vi "Generate BER Curve.vi"(4 "M-PSK":i32=4, 6 "Sample Step":dbl=0.3, 7 "Samples":i32=16, 9 "Message Bits":i32=2000, 10 "Synchronization Sequence":i32=20, 11 "Zero Pad":i32=16) -> (0 "error out":errorcluster, 3 "BER Curve":dbl[](array[numeric]))   [LabVIEW 2013]
uses:
  <vilib>/addons/Modulation/Digital/General/MT Generate Bits (Galois, PN Order).vi
  <vilib>/addons/Modulation/Digital/General/MT Generate PSK System Parameters(M).vi
  <vilib>/addons/Modulation/Digital/General/MT Generate PSK Synchronization Parameters (bit array).vi
  <vilib>/addons/Modulation/niDMT.lvlib
panel:
  out "O":bool[](array[boolean])
  out "I":bool[](array[boolean])
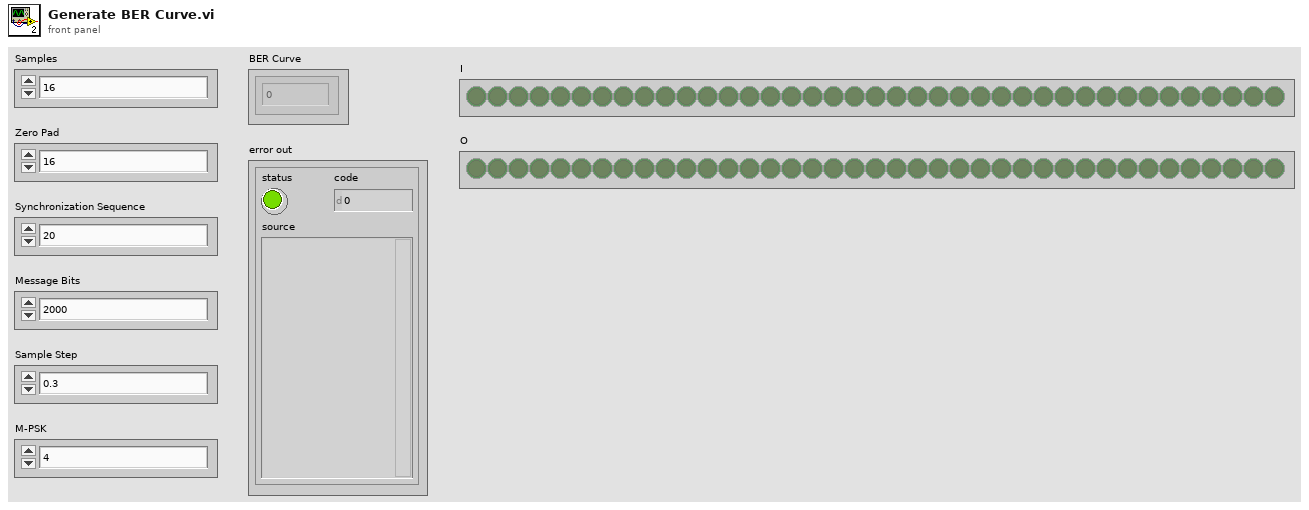
[diagram p1: front panel]
types:
  T1 = enum16{"FSK", "PSK", "QAM", "MSK", "PAM", "ASK", "CPM"}
  T2 = enum16{"none", "Raised Cosine", "Root Raised Cos", "Gaussian"}
  T3 = cluster{"samples per symbol (16)":i32, "symbol map":cdb[], "differential PSK":enum16{"disable", "enable"}, "PSK type":u16}
  T4 = typedef "niAMT.lvlib/Complex Data Waveform.ctl" = cluster{"t0":dbl, "dt":dbl, "Y":cdb[]}
  T5 = cluster{"expected sync location (symbols)":i32, "sync sequence":cdb[], "sync location uncertainty (symbols)":i32, "sync indent (symbols)":i32}
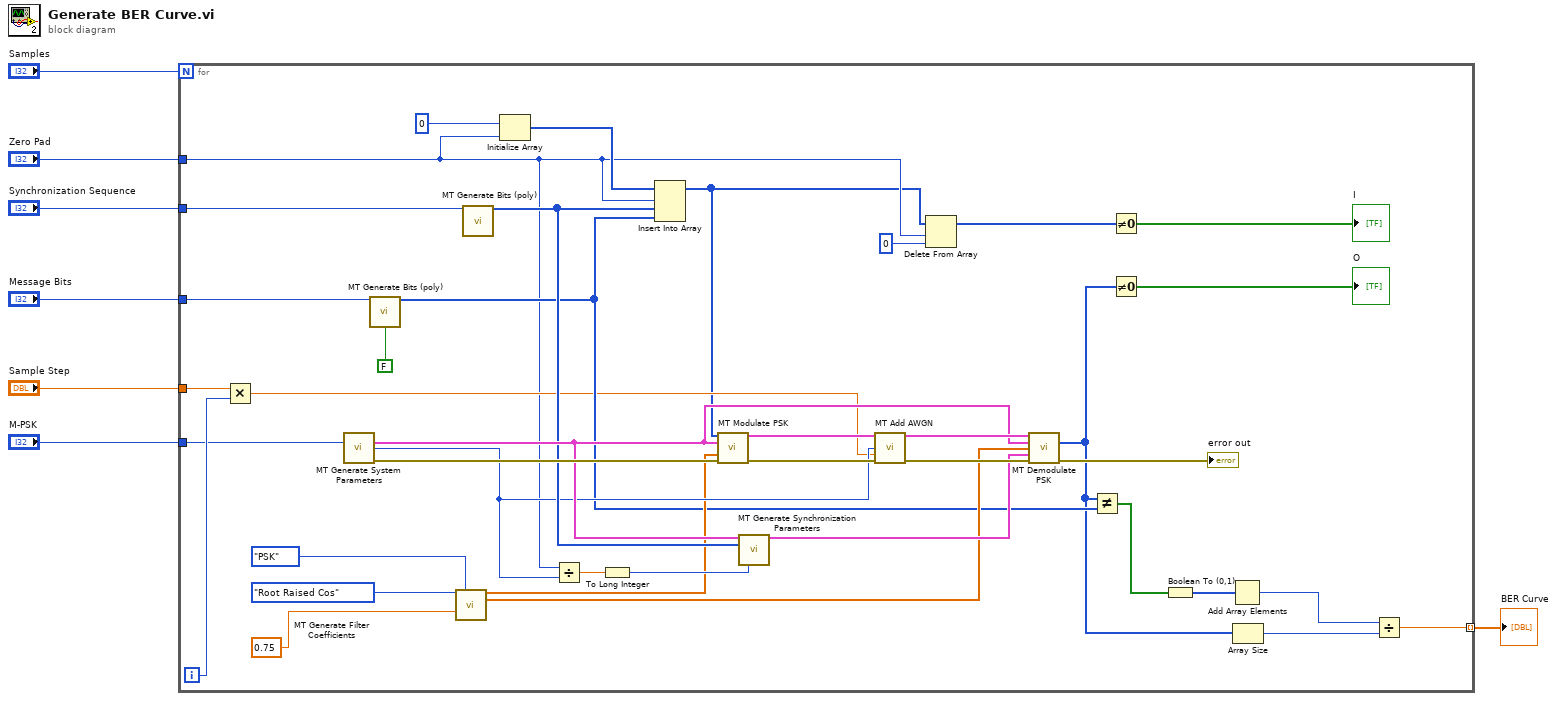
[diagram p0: block diagram]
diagram:
  n1 = for {
    N: "Samples" -> [_]
    tunnel: "Sample Step" -> [w20]
    tunnel: "Synchronization Sequence" -> [w19]
    tunnel: "Zero Pad" -> [w11]
    tunnel: "M-PSK" -> [w18]
    tunnel: [w17] -> w7 mode=indexing
    tunnel: "Message Bits" -> [w15]
    i -> [w21]
    n2 = Multiply(x=w20, y=w21) -> (x*y=w22:dbl)
    n3 = call-poly <vilib>:"MT Generate System Parameters.vi"("M-PSK (4)"=w18) -> ("PSK system parameters"=w38:T3, "bits per symbol"=w33:i32, "error out"=w43:errorcluster)  [unwired: 12 in]
    n4 = call-poly <vilib>:"MT Generate Bits (poly).vi"("total bits (128)"=w15, "reset? (T)"=FALSE) -> ("output bit stream"=w23:i8[])  [unwired: 11 in, 2 out]
    n5 = call <vilib>:"MT Generate Filter Coefficients.vi"("pulse shaping filter (none)"=T2."Root Raised Cos", "modulation type"=T1."PSK", "filter parameter"=0.75) -> ("pulse shaping filter coefficients"=w32:dbl[], "matched filter coefficients"=w31:dbl[])  [unwired: 10 in, 1 out]
    n6 = call-poly <vilib>:"MT Generate Bits (poly).vi"("total bits (128)"=w19) -> ("output bit stream"=w34:i8[])  [unwired: 12 in, 2 out]
    n7 = Initialize Array "Initialize Array"(0, w11) -> (w45:i32[])
    n8 = Divide(x=w11, y=w33) -> (x/y=w36:dbl)
    n9 = To Long Integer(number=w36) -> (32bit integer=w35:i32)
    n10 = Insert Into Array "Insert Into Array"(array=w45, index=w11, new element #1=w34, new element #2=w23) -> (w10:i32[])
    n11 = call <vilib>:"MT Modulate PSK.vi"("input bit stream"=w10, "PSK system parameters"=w38, "pulse shaping filter coefficients"=w32, "error in (no error)"=w43) -> ("output complex waveform"=w42:T4, "error out"=w41:errorcluster)  [unwired: 9 in, 1 out]
    n12 = call-poly <vilib>:"MT Generate Synchronization Parameters.vi"("PSK system parameters"=w38, "sync bits"=w34, "expected sync location (symbols)"=w35) -> ("PSK synchronization parameters"=w37:T5)  [unwired: 11 in, 1 out]
    n13 = call <vilib>:"MT Add AWGN.vi"("input complex waveform"=w42, "bits per symbol (1)"=w33, "Eb/N0 (10 dB)"=w22, "error in (no error)"=w41) -> ("output complex waveform"=w39:T4, "error out"=w40:errorcluster)  [unwired: 9 in, 1 out]
    n14 = Delete From Array "Delete From Array"(array=w10, length=w11, index=0) -> (array with subset deleted=w14:i32[])  [unwired: 1 out]
    n15 = call <vilib>:"MT Demodulate PSK.vi"("input complex waveform"=w39, "PSK system parameters"=w38, "matched filter coefficients"=w31, "synchronization parameters"=w37, "error in (no error)"=w40) -> ("output bit stream"=w8:i8[], "error out"=→"error out":errorcluster)  [unwired: 6 in, 3 out]
    n16 = Not Equal?(x=w8, y=w23) -> (x != y?=w26:bool[])
    n17 = Not Equal To 0?(x=w14) -> (x != 0?=→"I":bool[])
    n18 = Not Equal To 0?(x=w8) -> (x != 0?=→"O":bool[])
    n19 = Boolean To (0,1)(Boolean=w26) -> (0, 1=w25:i16[])
    n20 = Add Array Elements(numeric array=w25) -> (sum=w28:i16)
    n21 = Array Size(array=w8) -> (size(s)=w27:i32)
    n22 = Divide(x=w28, y=w27) -> (x/y=w17:dbl)
  }
  "BER Curve" <- w7
